vi "rqcBob Window Config.vi"(0 "rqcBob in":refnum<class "rqcBob.lvclass">, 5 "Window.Open":u16, 7 "Window.Close":u16=3000, 11 "error in (no error)":errorcluster) -> (4 "rqcBob out":refnum<class "rqcBob.lvclass">, 15 "error out":errorcluster)   [LabVIEW 2018, in "rqcBob.lvclass"]
uses:
  rqcBob.lvclass
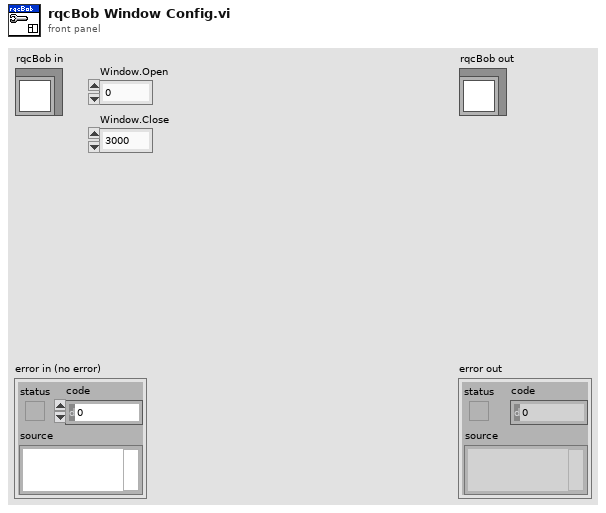
[diagram p1: front panel]
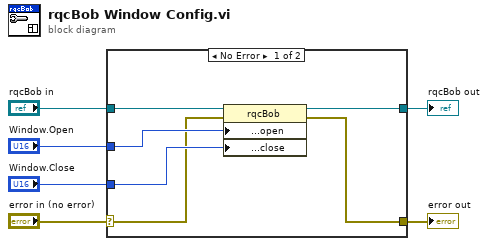
[diagram p0: block diagram]
diagram:
  n1 = case shown="No Error" "error in (no error)" {
    selector: "error in (no error)" -> [w8 w14]
    tunnel: [w7 w14] -> w5
    tunnel: [w11 w13] -> w3
    tunnel: "rqcBob in" -> [w12 w13]
    tunnel: "Window.Open" -> [w10 _]
    tunnel: "Window.Close" -> [w9 _]
    frame No Error {
      n2 = property class="rqcBob"(reference=w12, error in=w8, "public:Public Properties Access:Window:window.open"=w10, "public:Public Properties Access:Window:window.close"=w9) -> (reference out=w11:refnum<class "rqcBob.lvclass">, error out=w7:errorcluster)
    }
    frame Error {
    }
  }
  "error out" <- w5
  "rqcBob out" <- w3
